vi "Cycle 0 Coast to Zero.vi"(0 "GEA2 Reference In":refnum<k24>, 5 "GEA Inputs":T1 {"Destination" format="%.0x"; "Source" format="%.0x"}, 7 "Standalone?":bool, 11 "Error In":errorcluster) -> (4 "GEA2 Reference Out":refnum<k24>, 6 "Pass/Fail?":bool, 8 "Report Text":string, 15 "Error Out":errorcluster)   [LabVIEW 2016, in "TLMB.lvlib"]
uses:
  Projects/TLMB.lvlib
  Q:/Common/DLLs/GEA3/GeaCommunication.dll
  Common/DLLs/GEA3/GeaCommunication.dll
  Common/LabVIEW GEA2 Toolkit/LabVIEW_GEA2_Toolkit.lvlibp/type defs/Source_Destination.ctl
  TLMB Common/type defs/Drive Cycle Engine Request State.ctl
  Common/LabVIEW GEA2 Toolkit/LabVIEW_GEA2_Toolkit.lvlibp/type defs/ERD Read Data In.ctl
  Common/LabVIEW GEA2 Toolkit/LabVIEW_GEA2_Toolkit.lvlibp/type defs/Data Type.ctl
  Common/LabVIEW GEA2 Toolkit/LabVIEW_GEA2_Toolkit.lvlibp
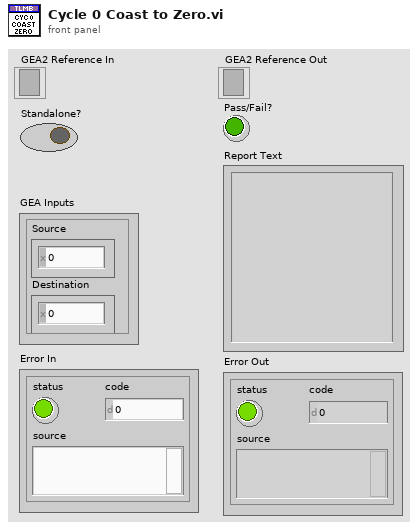
[diagram p1: front panel]
types:
  T1 = typedef "LabVIEW_GEA2_Toolkit.lvlibp/Source_Destination.ctl" = cluster{"Source":u8, "Destination":u8}
  T2 = typedef "TLMB.lvlib/Drive Cycle Engine Request State.ctl" = enum16{"Start", "Stop", "Pause", "Resume", "Select"}
  T3 = typedef "LabVIEW_GEA2_Toolkit.lvlibp/ERD Read Data In.ctl" = cluster{"ERD Number":u16, "Data Type":T4}
  T4 = typedef "LabVIEW_GEA2_Toolkit.lvlibp/Data Type.ctl" = enum16{"string", "boolean", "uint8_t", "uint16_t", "uint32_t", "uint64_t", "int8_t", "int16_t", "int32_t", "int64_t"}
  T5 = typedef "LabVIEW_GEA2_Toolkit.lvlibp/ERD Read Data Out.ctl" = cluster{"ERD Number":u16, "Data":string}
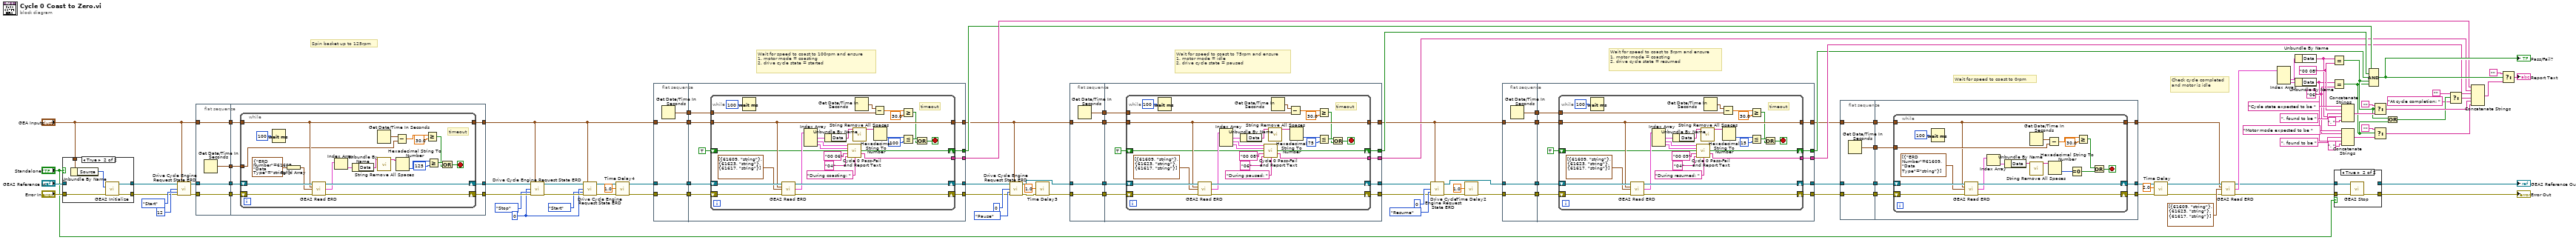
[diagram p0: block diagram]
diagram:
  w86 = "00 0B" ("y")
  w76 = "06" ("y")
  w99 = u8 0 ("Cycle ID")
  # "Check cycle completed\nand motor is idle"
  # "Wait for speed to coast to 0rpm"
  # "Wait for speed to coast to 5rpm and ensure\n1. motor mode = coasting\n2. drive cycle state = resumed"
  # "Wait for speed to coast to 75rpm and ensure\n1. motor mode = idle\n2. drive cycle state = paused"
  # "Wait for speed to coast to 100rpm and ensure\n1. motor mode = coasting\n2. drive cycle state = started"
  # "Spin basket up to 125rpm"
  n1 = case shown="True" "Standalone?" {
    tunnel: "GEA2 Reference In" -> [w110 _]
    tunnel: [w110 w115] -> w28
    tunnel: "Error In" -> [w109 w114]
    tunnel: [w109 w113] -> w26
    tunnel: "GEA Inputs" -> [_ w112]
    frame False {
    }
    frame True {
      n2 = Unbundle By Name(w112) -> ("Source"=w111:u8)
      n3 = call "GEA2 Initialize.vi"("Source Address"=w111, "error in"=w114) -> ("GEA2 Reference Out"=w115:refnum<k24>, "error out"=w113:errorcluster)  [unwired: 11 in, 1 out]
    }
  }
  n4 = call "Drive Cycle Engine Request State ERD.vi"("GEA2 Reference In"=w28, "GEA Inputs"="GEA Inputs", "Cycle ID"=u8 12, "Drive Cycle Engine Request State"=Drive_Cycle_Engine_Request_State."Start", "Error In"=w26) -> ("GEA2 Reference Out"=w105:refnum<k24>, "Error Out"=w106:errorcluster)  [unwired: 9 in]
  n5 = flat-sequence {
    tunnel: "GEA Inputs" -> [w117]
    tunnel: w105 -> [w118]
    tunnel: w106 -> [w119]
    tunnel: [w119] -> w97
    tunnel: [w118] -> w96
    tunnel: [w117] -> w95
    tunnel: [w116] -> w94
    tunnel: [w124] -> w104
    tunnel: [w123] -> w103
    tunnel: [w121] -> w56
    tunnel: w97 -> [w126]
    tunnel: w96 -> [w125]
    tunnel: w95 -> [w122]
    tunnel: w94 -> [w120]
    frame #0 {
      n6 = Get Date/Time In Seconds() -> (seconds since 1Jan1904=w116:timestamp)
    }
    frame #1 {
      n7 = while {
        shift-right: [w146] -> w123
        shift-left: w126 -> [w147]
        shift-right: [w144] -> w124
        shift-left: w125 -> [w145]
        tunnel: w122 -> [w137]
        tunnel: [w137] -> w121
        tunnel: w120 -> [w135]
        stop <- w132 stop-if-true
        # "timeout"
        n8 = Wait (ms)(milliseconds to wait=u32 100) -> ()  [unwired: 1 out]
        n9 = Build Array(T3 {"ERD Number"=61609, "Data Type"=enum."string"} ("ERD Read Data In")) -> (w143:T3[])
        n10 = call "GEA2 Read ERD.vi"("GEA2 Reference In"=w145, "GEA Inputs"=w137, "Read ERD List"=w143, "Error In"=w147) -> ("GEA2 Reference Out"=w144:refnum<k24>, "ERD Data Out"=w141:T5[], "Error Out"=w146:errorcluster)  [unwired: 8 in, 1 out]
        n11 = Index Array(array=w141) -> (element=w140:T5)  [unwired: 1 in]
        n12 = Unbundle By Name(w140) -> ("Data"=w127:string)
        n13 = Get Date/Time In Seconds() -> (seconds since 1Jan1904=w136:timestamp)
        n14 = call "String Remove All Spaces.vi"("Input String"=w127) -> ("Spaces Removed"=w128:string)  [unwired: 13 in, 1 out]
        n15 = Subtract(x=w136, y=w135) -> (x-y=w134:dbl)
        n16 = Hexadecimal String To Number(string=w128) -> (number=w139:u32)  [unwired: 2 in, 1 out]
        n17 = Greater Or Equal?(x=w134, y=30.0) -> (x >= y?=w130:bool)
        n18 = Greater Or Equal?(x=w139, y=u32 125) -> (x >= y?=w131:bool)
        n19 = Or(x=w131, y=w130) -> (x .or. y?=w132:bool)
      }
    }
  }
  n20 = call "Drive Cycle Engine Request State ERD.vi"("GEA2 Reference In"=w104, "GEA Inputs"=w56, "Cycle ID"=w99, "Drive Cycle Engine Request State"=Drive_Cycle_Engine_Request_State."Stop", "Error In"=w103) -> ("GEA2 Reference Out"=w101:refnum<k24>, "Error Out"=w100:errorcluster)  [unwired: 9 in]
  n21 = call "Drive Cycle Engine Request State ERD.vi"("GEA2 Reference In"=w101, "GEA Inputs"=w56, "Cycle ID"=w99, "Drive Cycle Engine Request State"=Drive_Cycle_Engine_Request_State."Start", "Error In"=w100) -> ("GEA2 Reference Out"=w57:refnum<k24>, "Error Out"=w2:errorcluster)  [unwired: 9 in]
  n22 = call "Time Delay4"("error in (no error)"=w2, "Delay Time (s)"=1.0) -> ("error out"=w1:errorcluster)  [unwired: 9 in]
  n23 = flat-sequence {
    tunnel: w1 -> [w149]
    tunnel: w56 -> [w150]
    tunnel: w57 -> [w151]
    tunnel: [w151] -> w61
    tunnel: [w150] -> w60
    tunnel: [w149] -> w59
    tunnel: [w148] -> w58
    tunnel: w61 -> [w161]
    tunnel: w60 -> [w160]
    tunnel: w59 -> [w159]
    tunnel: w58 -> [w158]
    tunnel: [w156] -> w54
    tunnel: [w155] -> w55
    tunnel: [w154] -> w46
    tunnel: [w153] -> w52
    tunnel: [w152] -> w53
    frame #0 {
      n24 = Get Date/Time In Seconds() -> (seconds since 1Jan1904=w148:timestamp)
    }
    frame #1 {
      n25 = while {
        shift-right: [w188] -> w156
        shift-left: w159 -> [w189]
        shift-right: [w186] -> w155
        shift-left: w161 -> [w187]
        tunnel: w160 -> [w183]
        tunnel: [w183] -> w154
        tunnel: w158 -> [w180]
        shift-right: [w166] -> w153
        shift-left: TRUE -> [w167]
        tunnel: [w165] -> w152
        stop <- w177 stop-if-true
        # "timeout"
        n26 = Wait (ms)(milliseconds to wait=u32 100) -> ()  [unwired: 1 out]
        n27 = call "GEA2 Read ERD.vi"("GEA2 Reference In"=w187, "GEA Inputs"=w183, "Read ERD List"=T3[] [{"ERD Number"=61609, "Data Type"=enum."string"}, {"ERD Number"=61623, "Data Type"=enum."string"}, {"ERD Number"=61617, "Data Type"=enum."string"}], "Error In"=w189) -> ("GEA2 Reference Out"=w186:refnum<k24>, "ERD Data Out"=w185:T5[], "Error Out"=w188:errorcluster)  [unwired: 8 in, 1 out]
        n28 = Index Array(array=w185) -> (element #1=w184:T5, element #2=w169:T5, element #3=w168:T5)  [unwired: 3 in]
        n29 = Unbundle By Name(w184) -> ("Data"=w172:string)
        n30 = call "Cycle 0 Pass-Fail and Report Text.vi"("Drive Cycle State"=w169, "Motor Mode"=w168, "Previous Pass/Fail"=w167, "Cycle State Expected"="00 06", "Motor Mode Expected"="04", "Header"="During coasting: ") -> ("Pass/Fail?"=w166:bool, "Report Text"=w165:string)  [unwired: 8 in]
        n31 = call "String Remove All Spaces.vi"("Input String"=w172) -> ("Spaces Removed"=w173:string)  [unwired: 13 in, 1 out]
        n32 = Get Date/Time In Seconds() -> (seconds since 1Jan1904=w179:timestamp)
        n33 = Subtract(x=w179, y=w180) -> (x-y=w181:dbl)
        n34 = Hexadecimal String To Number(string=w173) -> (number=w171:u32)  [unwired: 2 in, 1 out]
        n35 = Greater Or Equal?(x=w181, y=30.0) -> (x >= y?=w176:bool)
        n36 = Less Or Equal?(x=w171, y=u32 100) -> (x <= y?=w178:bool)
        n37 = Or(x=w178, y=w176) -> (x .or. y?=w177:bool)
      }
    }
  }
  n38 = call "Drive Cycle Engine Request State ERD.vi"("GEA2 Reference In"=w55, "GEA Inputs"=w46, "Cycle ID"=u8 0, "Drive Cycle Engine Request State"=Drive_Cycle_Engine_Request_State."Pause", "Error In"=w54) -> ("GEA2 Reference Out"=w47:refnum<k24>, "Error Out"=w5:errorcluster)  [unwired: 9 in]
  n39 = call "Time Delay3"("error in (no error)"=w5, "Delay Time (s)"=1.0) -> ("error out"=w4:errorcluster)  [unwired: 9 in]
  n40 = flat-sequence {
    tunnel: w4 -> [w191]
    tunnel: w46 -> [w192]
    tunnel: w47 -> [w193]
    tunnel: [w193] -> w51
    tunnel: [w192] -> w50
    tunnel: [w191] -> w49
    tunnel: [w190] -> w48
    tunnel: w51 -> [w203]
    tunnel: w50 -> [w202]
    tunnel: w49 -> [w201]
    tunnel: w48 -> [w200]
    tunnel: [w198] -> w43
    tunnel: [w197] -> w44
    tunnel: [w196] -> w37
    tunnel: [w195] -> w45
    tunnel: [w194] -> w30
    frame #0 {
      n41 = Get Date/Time In Seconds() -> (seconds since 1Jan1904=w190:timestamp)
    }
    frame #1 {
      n42 = while {
        shift-right: [w230] -> w198
        shift-left: w201 -> [w231]
        shift-right: [w228] -> w197
        shift-left: w203 -> [w229]
        tunnel: w202 -> [w225]
        tunnel: [w225] -> w196
        tunnel: w200 -> [w222]
        shift-right: [w208] -> w195
        shift-left: TRUE -> [w209]
        tunnel: [w207] -> w194
        stop <- w219 stop-if-true
        # "timeout"
        n43 = Wait (ms)(milliseconds to wait=u32 100) -> ()  [unwired: 1 out]
        n44 = call "GEA2 Read ERD.vi"("GEA2 Reference In"=w229, "GEA Inputs"=w225, "Read ERD List"=T3[] [{"ERD Number"=61609, "Data Type"=enum."string"}, {"ERD Number"=61623, "Data Type"=enum."string"}, {"ERD Number"=61617, "Data Type"=enum."string"}], "Error In"=w231) -> ("GEA2 Reference Out"=w228:refnum<k24>, "ERD Data Out"=w227:T5[], "Error Out"=w230:errorcluster)  [unwired: 8 in, 1 out]
        n45 = Index Array(array=w227) -> (element #1=w226:T5, element #2=w211:T5, element #3=w210:T5)  [unwired: 3 in]
        n46 = Unbundle By Name(w226) -> ("Data"=w214:string)
        n47 = call "Cycle 0 Pass-Fail and Report Text.vi"("Drive Cycle State"=w211, "Motor Mode"=w210, "Previous Pass/Fail"=w209, "Cycle State Expected"="00 08", "Motor Mode Expected"="06", "Header"="During paused: ") -> ("Pass/Fail?"=w208:bool, "Report Text"=w207:string)  [unwired: 8 in]
        n48 = call "String Remove All Spaces.vi"("Input String"=w214) -> ("Spaces Removed"=w215:string)  [unwired: 13 in, 1 out]
        n49 = Get Date/Time In Seconds() -> (seconds since 1Jan1904=w221:timestamp)
        n50 = Subtract(x=w221, y=w222) -> (x-y=w223:dbl)
        n51 = Hexadecimal String To Number(string=w215) -> (number=w213:u32)  [unwired: 2 in, 1 out]
        n52 = Greater Or Equal?(x=w223, y=30.0) -> (x >= y?=w218:bool)
        n53 = Less Or Equal?(x=w213, y=u32 75) -> (x <= y?=w220:bool)
        n54 = Or(x=w220, y=w218) -> (x .or. y?=w219:bool)
      }
    }
  }
  n55 = call "Drive Cycle Engine Request State ERD.vi"("GEA2 Reference In"=w44, "GEA Inputs"=w37, "Cycle ID"=u8 0, "Drive Cycle Engine Request State"=Drive_Cycle_Engine_Request_State."Resume", "Error In"=w43) -> ("GEA2 Reference Out"=w38:refnum<k24>, "Error Out"=w8:errorcluster)  [unwired: 9 in]
  n56 = call "Time Delay2"("error in (no error)"=w8, "Delay Time (s)"=1.0) -> ("error out"=w7:errorcluster)  [unwired: 9 in]
  n57 = flat-sequence {
    tunnel: w7 -> [w233]
    tunnel: w37 -> [w234]
    tunnel: w38 -> [w235]
    tunnel: [w235] -> w42
    tunnel: [w234] -> w41
    tunnel: [w233] -> w40
    tunnel: [w232] -> w39
    tunnel: w42 -> [w245]
    tunnel: w41 -> [w244]
    tunnel: w40 -> [w243]
    tunnel: w39 -> [w242]
    tunnel: [w240] -> w33
    tunnel: [w239] -> w34
    tunnel: [w238] -> w32
    tunnel: [w237] -> w35
    tunnel: [w236] -> w36
    frame #0 {
      n58 = Get Date/Time In Seconds() -> (seconds since 1Jan1904=w232:timestamp)
    }
    frame #1 {
      n59 = while {
        shift-right: [w272] -> w240
        shift-left: w243 -> [w273]
        shift-right: [w270] -> w239
        shift-left: w245 -> [w271]
        tunnel: w244 -> [w267]
        tunnel: [w267] -> w238
        tunnel: w242 -> [w264]
        shift-right: [w250] -> w237
        shift-left: TRUE -> [w251]
        tunnel: [w249] -> w236
        stop <- w261 stop-if-true
        # "timeout"
        n60 = Wait (ms)(milliseconds to wait=u32 100) -> ()  [unwired: 1 out]
        n61 = call "GEA2 Read ERD.vi"("GEA2 Reference In"=w271, "GEA Inputs"=w267, "Read ERD List"=T3[] [{"ERD Number"=61609, "Data Type"=enum."string"}, {"ERD Number"=61623, "Data Type"=enum."string"}, {"ERD Number"=61617, "Data Type"=enum."string"}], "Error In"=w273) -> ("GEA2 Reference Out"=w270:refnum<k24>, "ERD Data Out"=w269:T5[], "Error Out"=w272:errorcluster)  [unwired: 8 in, 1 out]
        n62 = Index Array(array=w269) -> (element #1=w268:T5, element #2=w253:T5, element #3=w252:T5)  [unwired: 3 in]
        n63 = Unbundle By Name(w268) -> ("Data"=w256:string)
        n64 = call "Cycle 0 Pass-Fail and Report Text.vi"("Drive Cycle State"=w253, "Motor Mode"=w252, "Previous Pass/Fail"=w251, "Cycle State Expected"="00 09", "Motor Mode Expected"="04", "Header"="During resumed: ") -> ("Pass/Fail?"=w250:bool, "Report Text"=w249:string)  [unwired: 8 in]
        n65 = call "String Remove All Spaces.vi"("Input String"=w256) -> ("Spaces Removed"=w257:string)  [unwired: 13 in, 1 out]
        n66 = Get Date/Time In Seconds() -> (seconds since 1Jan1904=w263:timestamp)
        n67 = Subtract(x=w263, y=w264) -> (x-y=w265:dbl)
        n68 = Hexadecimal String To Number(string=w257) -> (number=w255:u32)  [unwired: 2 in, 1 out]
        n69 = Greater Or Equal?(x=w265, y=30.0) -> (x >= y?=w260:bool)
        n70 = Less Or Equal?(x=w255, y=u32 15) -> (x <= y?=w262:bool)
        n71 = Or(x=w262, y=w260) -> (x .or. y?=w261:bool)
      }
    }
  }
  n72 = flat-sequence {
    tunnel: [w277] -> w71
    tunnel: w34 -> [w276]
    tunnel: [w276] -> w70
    tunnel: w33 -> [w275]
    tunnel: [w275] -> w69
    tunnel: w32 -> [w274]
    tunnel: [w274] -> w31
    tunnel: w71 -> [w284]
    tunnel: [w283] -> w11
    tunnel: [w282] -> w68
    tunnel: w70 -> [w281]
    tunnel: w69 -> [w280]
    tunnel: w31 -> [w279]
    tunnel: [w278] -> w19
    frame #0 {
      n73 = Get Date/Time In Seconds() -> (seconds since 1Jan1904=w277:timestamp)
    }
    frame #1 {
      n74 = while {
        shift-right: [w302] -> w283
        shift-left: w280 -> [w303]
        shift-right: [w300] -> w282
        shift-left: w281 -> [w301]
        tunnel: w284 -> [w295]
        tunnel: w279 -> [w285]
        tunnel: [w285] -> w278
        stop <- w293 stop-if-true
        n75 = Wait (ms)(milliseconds to wait=u32 100) -> ()  [unwired: 1 out]
        n76 = call "GEA2 Read ERD.vi"("GEA2 Reference In"=w301, "GEA Inputs"=w285, "Read ERD List"=T3[] [{"ERD Number"=61609, "Data Type"=enum."string"}], "Error In"=w303) -> ("GEA2 Reference Out"=w300:refnum<k24>, "ERD Data Out"=w299:T5[], "Error Out"=w302:errorcluster)  [unwired: 8 in, 1 out]
        n77 = Index Array(array=w299) -> (element=w298:T5)  [unwired: 1 in]
        n78 = Unbundle By Name(w298) -> ("Data"=w289:string)
        n79 = Get Date/Time In Seconds() -> (seconds since 1Jan1904=w294:timestamp)
        n80 = call "String Remove All Spaces.vi"("Input String"=w289) -> ("Spaces Removed"=w290:string)  [unwired: 13 in, 1 out]
        n81 = Subtract(x=w294, y=w295) -> (x-y=w296:dbl)
        n82 = Hexadecimal String To Number(string=w290) -> (number=w288:u32)  [unwired: 2 in, 1 out]
        n83 = Equal To 0?(x=w288) -> (x = 0?=w287:bool)
        n84 = Greater Or Equal?(x=w296, y=30.0) -> (x >= y?=w286:bool)
        n85 = Or(x=w286, y=w287) -> (x .or. y?=w293:bool)
      }
    }
  }
  n86 = call "Time Delay"("error in (no error)"=w11, "Delay Time (s)"=2.0) -> ("error out"=w10:errorcluster)  [unwired: 9 in]
  n87 = call "GEA2 Read ERD.vi"("GEA2 Reference In"=w68, "GEA Inputs"=w19, "Read ERD List"=T3[] [{"ERD Number"=61609, "Data Type"=enum."string"}, {"ERD Number"=61623, "Data Type"=enum."string"}, {"ERD Number"=61617, "Data Type"=enum."string"}], "Error In"=w10) -> ("GEA2 Reference Out"=w21:refnum<k24>, "ERD Data Out"=w90:T5[], "Error Out"=w23:errorcluster)  [unwired: 8 in, 1 out]
  n88 = Index Array(array=w90) -> (element #2=w93:T5, element #3=w92:T5)  [unwired: 3 in, 1 out]
  n89 = Unbundle By Name(w93) -> ("Data"=w84:string)
  n90 = Unbundle By Name(w92) -> ("Data"=w74:string)
  n91 = Equal?(x=w84, y=w86) -> (x = y?=w17:bool)
  n92 = Equal?(x=w74, y=w76) -> (x = y?=w16:bool)
  n93 = case shown="True" "Standalone?" {
    tunnel: [w304 w308] -> w24
    tunnel: w23 -> [w304 w307]
    tunnel: w21 -> [w305 w306]
    tunnel: [w305 _] -> w20
    frame False {
    }
    frame True {
      n94 = call "GEA2 Stop.vi"("GEA2 Reference In"=w306, "Error In"=w307) -> ("Error Out"=w308:errorcluster)  [unwired: 13 in]
    }
  }
  "GEA2 Reference Out" <- w20
  "Error Out" <- w24
  n95 = Concatenate Strings("Cycle state expected to be " ("string"), w86, ", found to be " ("string"), w84, ". " ("string")) -> (w82:string)
  n96 = Concatenate Strings("Motor mode expected to be " ("string"), w76, ", found to be " ("string"), w74, ". " ("string")) -> (w79:string)
  n97 = Compound Arithmetic op=AND(w52, w45, w35, w17, w16) -> (w89:bool)
  "Pass/Fail?" <- w89
  n98 = Select(t="", s=w17, f=w82) -> (s? t:f=w67:string)
  n99 = Select(t="", s=w16, f=w79) -> (s? t:f=w66:string)
  n100 = Or(x=w17, y=w16) -> (x .or. y?=w15:bool)
  n101 = Select(t="", s=w15, f="At cycle completion: " ("string")) -> (s? t:f=w18:string)
  n102 = Concatenate Strings(w53, w30, w36, w18, w67, w66) -> (w78:string)
  n103 = Select(t="", s=w89, f=w78) -> (s? t:f=→"Report Text":string)
